vi "Set Class control icon.vi"() -> ()   [LabVIEW 2020]
uses:
  <vilib>/LabVIEW Icon API/API_User Layer Data.ctl
  <vilib>/Utility/miscctls.llb/LVPoint32TypeDef.ctl
  <vilib>/picture/picture.llb/imagedata.ctl
  <vilib>/LabVIEW Icon API/LabVIEW Icon API.lvlib
panel:
  in  "Project Path":path
  in  "My Computer?":bool
  in  "Array":path[](array[path])
  in  "Path":path
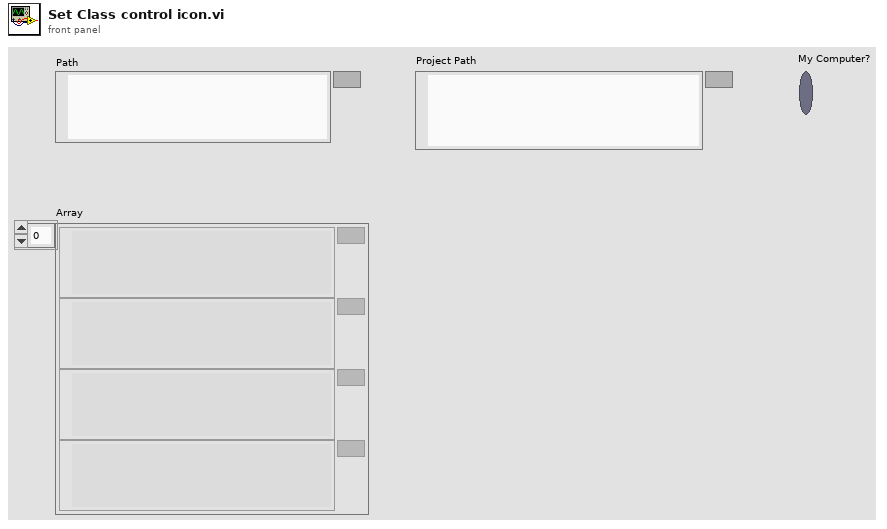
[diagram p1: front panel]
types:
  T1 = typedef "imagedata.ctl" = cluster{"image type":i32, "image depth":i32, "image":u8[], "mask":u8[], "colors":u32[], "Rectangle":cluster{"left":i16, "top":i16, "right":i16, "bottom":i16}}
  T2 = typedef "LabVIEW Icon API.lvlib/API_User Layer Data.ctl" = cluster{"Layer name":string, "Origin":T3, "Icon image data":T1}
  T3 = typedef "LVPoint32TypeDef.ctl" = cluster{"Horizontal":i32, "Vertical":i32}
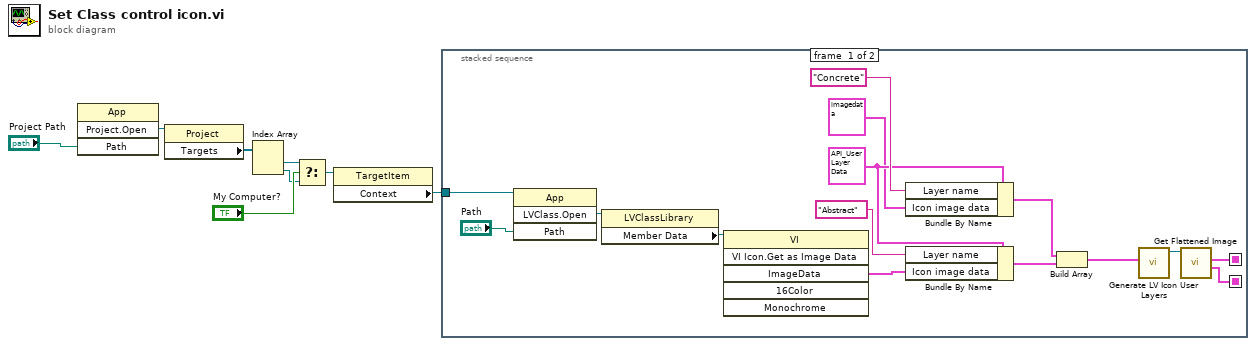
[diagram p0: block diagram]
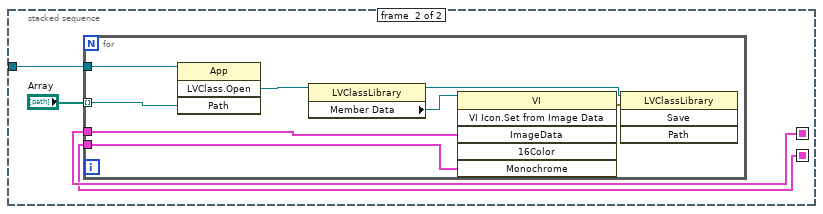
[diagram p2: hidden frame]
diagram:
  n1 = invoke class="App" method="Project.Open"("Path"="Project Path") -> ("Project:Open"=w8:refnum<vi>)  [unwired: 3 in, 3 out]
  n2 = property class="Project"(reference=w8) -> ("Targets"=w7:refnum<vi>[])  [unwired: 1 in, 2 out]
  n3 = Index Array(array=w7) -> (element #1=w4:refnum<vi>, element #2=w3:refnum<vi>)  [unwired: 2 in]
  n4 = Select(t=w4, s="My Computer?", f=w3) -> (s? t:f=w2:refnum<vi>)
  n5 = property class="TargetItem"(reference=w2) -> ("Context"=w1:refnum<vi>)  [unwired: 1 in, 2 out]
  n6 = stacked-sequence {
    seq-local: [w11 _] -> [_ w25]
    seq-local: [w10 _] -> [_ w24]
    tunnel: w1 -> [w20 w26]
    frame #0 {
      w14 = T2 {"Layer name"="", "Origin"={"Horizontal"=0, "Vertical"=0}, "Icon image data"={"image type"=0, "image depth"=0, "image"=[], "mask"=[], "colors"=[], "Rectangle"={"left"=0, "top"=0, "right"=0, "bottom"=0}}} ("User layer")
      n7 = invoke class="App" method="LVClass.Open"(reference=w20, "Path"="Path") -> ("LVClass.Open"=w22:refnum<vi>)  [unwired: 2 in, 3 out]
      n8 = property class="LVClassLibrary"(reference=w22) -> ("Member Data"=w21:refnum<vi>)  [unwired: 1 in, 2 out]
      n9 = invoke class="VI" method="VI Icon.Get as Image Data"(reference=w21) -> ("ImageData"=w19:T1)  [unwired: 5 in, 5 out]
      n10 = Bundle By Name(cluster=w14, "Layer name"="Concrete", "Icon image data"=T1 {"image type"=0, "image depth"=24, "image"=array[3072 elements], "mask"=[0, 0, 0, 0, 0, 0, 0, 0, 0, 0, 0, 0, 0, 0, 0, 0, 0, 0, 0, 0, 0, 0, 0, 0, 0, 0, 0, 0, 0, 0, 0, 0, 0, 0, 0, 0, 0, 0, 0, 0, 0, 0, 0, 0, 0, 0, 0, 0, 0, 0, 0, 0, 0, 0, 0, 0, 0, 0, 0, 0, 0, 0, 0, 0, 0, 0, 0, 0, 0, 0, 0, 0, 0, 0, 0, 0, 7, 248, 0, 0, 8, 56, 0, 0, 16, 120, 0, 0, 63, 248, 0, 0, 63, 248, 0, 0, 63, 248, 0, 0, 63, 248, 0, 0, 63, 248, 0, 0, 63, 240, 0, 0, 63, 224, 0, 0, 63, 192, 0, 0, 0, 0, 0, 0, 0, 0, 0, 0], "colors"=[], "Rectangle"={"left"=0, "top"=0, "right"=32, "bottom"=32}} ("Color Image")) -> (w16:T2)
      n11 = Bundle By Name(cluster=w14, "Layer name"="Abstract", "Icon image data"=w19) -> (w15:T2)
      n12 = Build Array(w16, w15) -> (w13:T2[])
      n13 = call <vilib>:"Generate LV Icon User Layers.vi"("User layers"=w13) -> ("Icon out"=w12:refnum<class "Icon.lvclass">)  [unwired: 9 in, 1 out]
      n14 = call <vilib>:"Get Flattened Image.vi"("lv_icon.lvlib:Icon.lvclass in"=w12) -> ("BW Image"=w10:T1, "Color Image"=w11:T1)  [unwired: 7 in, 2 out]
    }
    frame #1 {
      n15 = for {
        tunnel: "Array" -> [w34] mode=indexing
        tunnel: w25 -> [w33]
        tunnel: w24 -> [w31]
        tunnel: w26 -> [w28]
        n16 = invoke class="App" method="LVClass.Open"(reference=w28, "Path"=w34) -> ("LVClass.Open"=w35:refnum<vi>)  [unwired: 2 in, 3 out]
        n17 = property class="LVClassLibrary"(reference=w35) -> (reference out=w29:refnum<vi>, "Member Data"=w32:refnum<vi>)  [unwired: 1 in, 1 out]
        n18 = invoke class="VI" method="VI Icon.Set from Image Data"(reference=w32, "ImageData"=w33, "Monochrome"=w31) -> (error out=w30:errorcluster)  [unwired: 3 in, 5 out]
        n19 = invoke class="LVClassLibrary" method="Save"(reference=w29, error in=w30) -> ()  [unwired: 2 in, 4 out]
      }
    }
  }
